vi "InitDrive.vi"   [LabVIEW 2019]
doc: "This VI initializes devices related directly to the drive subsystem."
uses:
  <vilib>/Rock Robotics/WPI/Solenoid/WPI_SolenoidChannel.ctl
  <vilib>/Rock Robotics/WPI/ThirdParty/Phoenix-LabVIEW/Motor Controller/Controls/CTRE_Phoenix_MotorControl_TalonFXInvertType.ctl
  <vilib>/Rock Robotics/WPI/ThirdParty/Phoenix-LabVIEW/Motor Controller/Controls/CTRE_Phoenix_MotorControl_NeutralMode.ctl
  <vilib>/Rock Robotics/WPI/ThirdParty/Phoenix-LabVIEW/Motor Controller/Controls/CTRE_Phoenix_MotorControl_SupplyCurrentLimitConfiguration.ctl
  <vilib>/Rock Robotics/WPI/ThirdParty/Phoenix-LabVIEW/Motor Controller/Controls/CTRE_Phoenix_MotorControl_FeedbackDevice_TalonFX.ctl
  <vilib>/Rock Robotics/WPI/Solenoid/WPI_SolenoidOpenDouble.vi
  refnums.vi
types:
  T1 = typedef "CTRE_Phoenix_MotorControl_TalonFXInvertType.ctl" = enum16{"Counter-Clockwise", "Clockwise"}
  T2 = typedef "CTRE_Phoenix_MotorControl_FeedbackDevice_TalonFX.ctl" = i8
  T3 = typedef "CTRE_Phoenix_MotorControl_SupplyCurrentLimitConfiguration.ctl" = cluster{"Enable?":bool, "Current Limit":dbl, "Threshold Current":dbl, "Threshold Time":dbl}
  T4 = typedef "CTRE_Phoenix_MotorControl_NeutralMode.ctl" = enum8{"EEPROMSetting", "Override to Coast", "Override to Brake"}
  T5 = typedef "WPI_SolenoidChannel.ctl" = enum8{"Solenoid 0", "Solenoid 1", "Solenoid 2", "Solenoid 3", "Solenoid 4", "Solenoid 5", "Solenoid 6", "Solenoid 7", "Invalid"}
  T6 = typedef "WPI_MotorControlDeviceRef.ctl" = cluster{"DeviceStatus":errorcluster, "Type":T7, "PWM":cluster{"PWM Channel":T8, "DeadBand":T9}, "CAN":cluster{"Device Number":u8, "SetOutput VI Ref":variant, "GetOutput VI Ref":variant, "Enable VI Ref":variant, "Disable VI Ref":variant, "Data":variant}, "Invert":bool, "DIO PWM":cluster{"PWM \"Enable\" Channel":T8, "DIOChannel":T10, "PWM Rate":dbl}}
  T7 = typedef "WPI_MotorControlType.ctl" = enum16{"PWM", "CAN", "DIO PWM"}
  T8 = typedef "FPGA_DIOPWMChannel.ctl" = enum8{"PWM 0", "PWM 1", "PWM 2", "PWM 3", "PWM 4", "PWM 5", "PWM 6", "PWM 7", "PWM 8", "PWM 9", "PWM MXP 0", "PWM MXP 1", "PWM MXP 2", "PWM MXP 3", "PWM MXP 4", "PWM MXP 5", "PWM MXP 6", "PWM MXP 7", "PWM MXP 8", "PWM MXP 9", "Invalid"}
  T9 = typedef "WPI_PWMDeadband.ctl" = cluster{"Name":string, "maxPositivePwm":i32, "minPositivePwm":i32, "centerPwm":i32, "maxNegativePwm":i32, "minNegativePwm":i32, "angularRange":u16}
  T10 = typedef "FPGA_DIOChannel.ctl" = enum8{"DIO 0", "DIO 1", "DIO 2", "DIO 3", "DIO 4", "DIO 5", "DIO 6", "DIO 7", "DIO 8", "DIO 9", "DIO MXP 0", "DIO MXP 1", "DIO MXP 2", "DIO MXP 3", "DIO MXP 4", "DIO MXP 5", "DIO MXP 6", "DIO MXP 7", "DIO MXP 8", "DIO MXP 9", "DIO MXP 10", "DIO MXP 11", "DIO MXP 12", "DIO MXP 13", "DIO MXP 14", "DIO MXP 15", "SPI Port CS1", "SPI Port CS2", "SPI Port CS3", "SPI Port MISO", "SPI Port MOSI", "Invalid"}
  T11 = typedef "WPI_SolenoidDevRef.ctl" = cluster{"DevStatus":errorcluster, "Pneumatics Control Module":u8, "Forward Solenoid Channel":T5, "Reverse Solenoid Channel":T5}
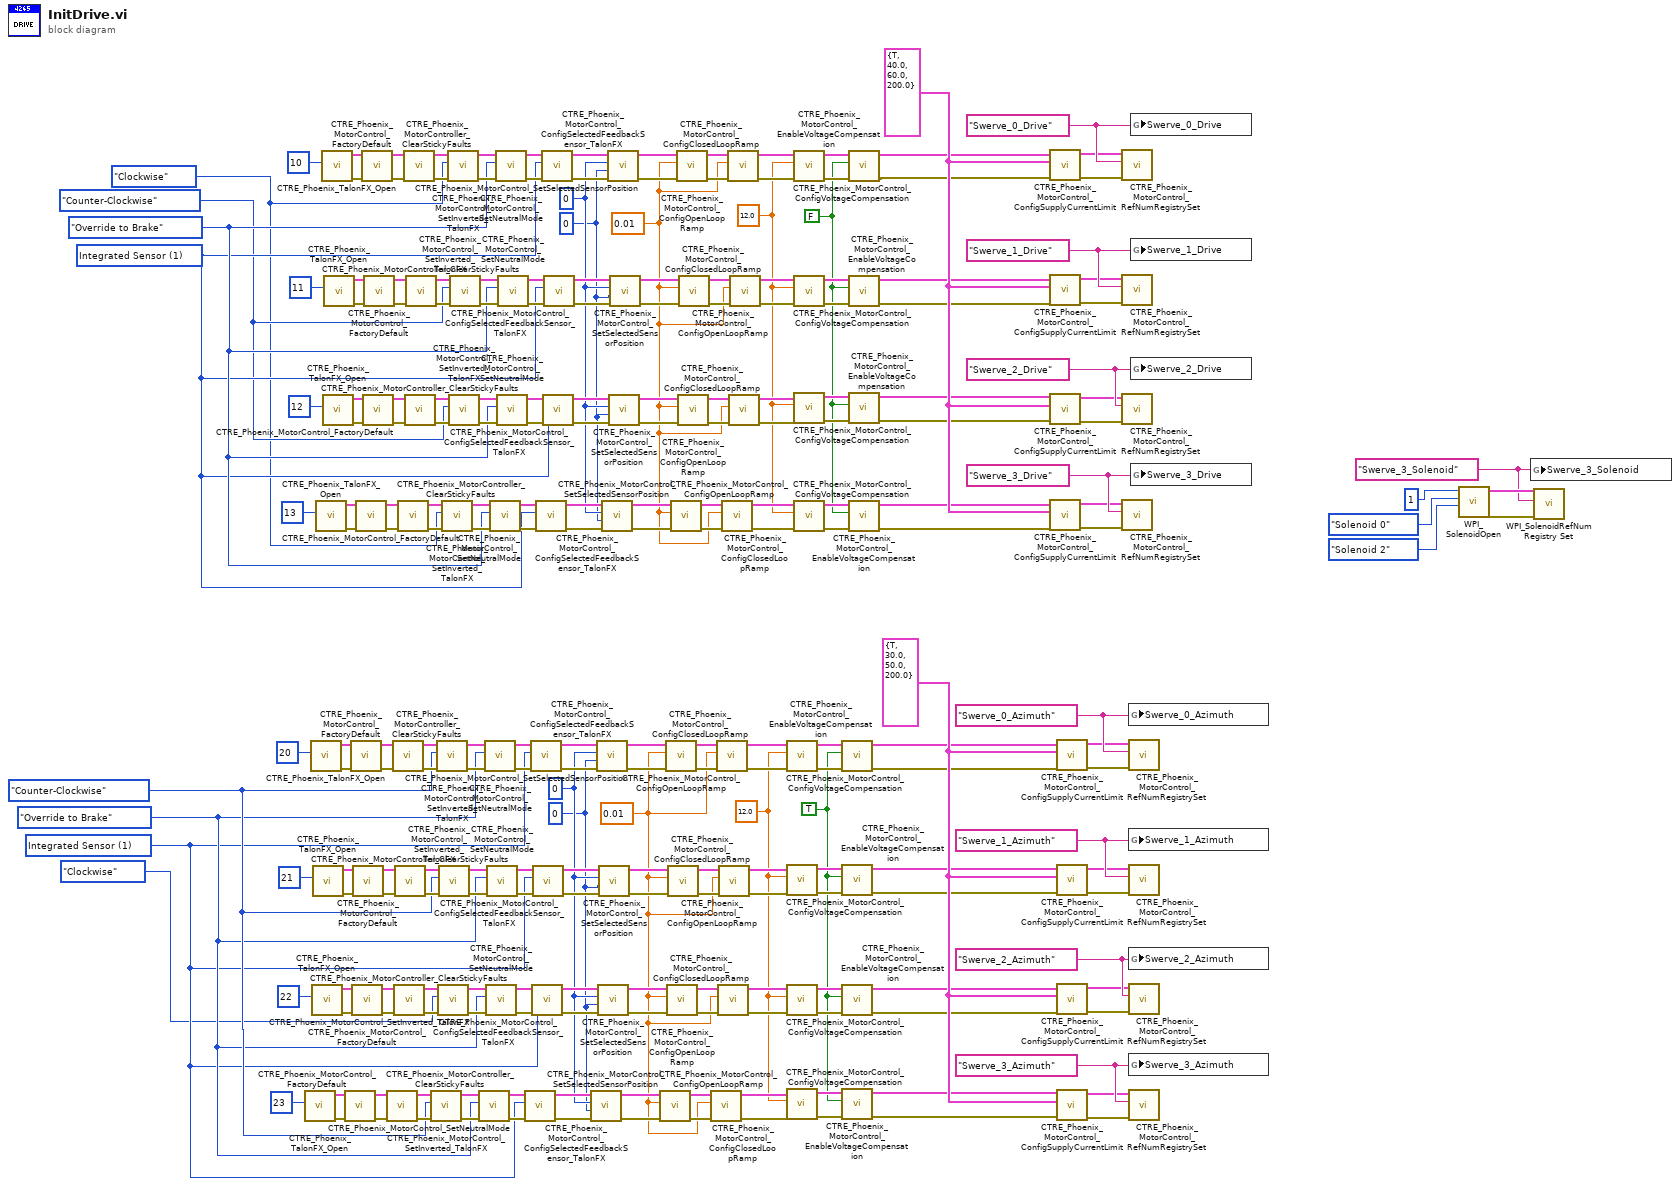
[diagram p0: block diagram]
diagram:
  w4 = CTRE_Phoenix_MotorControl_TalonFXInvertType."Clockwise" ("Invert Type")
  w6 = TRUE ("Enable Voltage Compensation?")
  w7 = 12.0 ("Saturation Voltage")
  w8 = FALSE ("Enable Voltage Compensation?")
  w9 = 12.0 ("Saturation Voltage")
  w56 = T2 1 items=["Integrated Sensor"=1, "Sensor Sum (S0 + S1)"=9, "Sensor Difference (D0 - D1)"=10, "Remote Source 0"=11, "Remote Source 1"=12, "None"=14, "Software Emulated"=15] ("Talon FX Feedback Device")
  w62 = T3 {"Enable?"=TRUE, "Current Limit"=30.0, "Threshold Current"=50.0, "Threshold Time"=200.0} ("Supply Current Limit Configuration")
  w57 = 0.01 ("secondsFromNeutralToFull")
  w58 = u32 0 ("pidLoopIdx")
  w59 = 0 ("New Sensor Position")
  w60 = CTRE_Phoenix_MotorControl_NeutralMode."Override to Brake" ("Motor Control Neutral Mode")
  w61 = CTRE_Phoenix_MotorControl_TalonFXInvertType."Counter-Clockwise" ("Invert Type")
  w78 = "Swerve_0_Azimuth" ("refnum name")
  w98 = "Swerve_1_Azimuth" ("refnum name")
  w118 = "Swerve_2_Azimuth" ("refnum name")
  w138 = "Swerve_3_Azimuth" ("refnum name")
  w146 = T2 1 items=["Integrated Sensor"=1, "Sensor Sum (S0 + S1)"=9, "Sensor Difference (D0 - D1)"=10, "Remote Source 0"=11, "Remote Source 1"=12, "None"=14, "Software Emulated"=15] ("Talon FX Feedback Device")
  w148 = T3 {"Enable?"=TRUE, "Current Limit"=40.0, "Threshold Current"=60.0, "Threshold Time"=200.0} ("Supply Current Limit Configuration")
  w143 = 0.01 ("secondsFromNeutralToFull")
  w144 = u32 0 ("pidLoopIdx")
  w145 = 0 ("New Sensor Position")
  w147 = CTRE_Phoenix_MotorControl_NeutralMode."Override to Brake" ("Motor Control Neutral Mode")
  w5 = CTRE_Phoenix_MotorControl_TalonFXInvertType."Counter-Clockwise" ("Invert Type")
  w164 = "Swerve_0_Drive" ("refnum name")
  w184 = "Swerve_1_Drive" ("refnum name")
  w204 = "Swerve_2_Drive" ("refnum name")
  w224 = "Swerve_3_Drive" ("refnum name")
  w229 = "Swerve_3_Solenoid" ("refnum name")
  n1 = call <vilib>:"CTRE_Phoenix_TalonFX_Open.vi"("Device Number"=u8 23 ("Drive 4L")) -> ("error out"=w127:errorcluster, "CAN Talon SRX Ref"=w134:T6)  [unwired: 9 in]
  n2 = call <vilib>:"CTRE_Phoenix_TalonFX_Open.vi"("Device Number"=u8 20 ("Drive 4L")) -> ("error out"=w67:errorcluster, "CAN Talon SRX Ref"=w74:T6)  [unwired: 9 in]
  n3 = call <vilib>:"CTRE_Phoenix_TalonFX_Open.vi"("Device Number"=u8 22 ("Drive 4L")) -> ("error out"=w107:errorcluster, "CAN Talon SRX Ref"=w114:T6)  [unwired: 9 in]
  n4 = call <vilib>:"CTRE_Phoenix_TalonFX_Open.vi"("Device Number"=u8 21 ("Drive 4L")) -> ("error out"=w87:errorcluster, "CAN Talon SRX Ref"=w94:T6)  [unwired: 9 in]
  n5 = call <vilib>:"CTRE_Phoenix_TalonFX_Open.vi"("Device Number"=u8 13 ("Drive 4L")) -> ("error out"=w213:errorcluster, "CAN Talon SRX Ref"=w220:T6)  [unwired: 9 in]
  n6 = call <vilib>:"CTRE_Phoenix_TalonFX_Open.vi"("Device Number"=u8 10 ("Drive 4L")) -> ("error out"=w153:errorcluster, "CAN Talon SRX Ref"=w160:T6)  [unwired: 9 in]
  n7 = call <vilib>:"CTRE_Phoenix_TalonFX_Open.vi"("Device Number"=u8 12 ("Drive 4L")) -> ("error out"=w193:errorcluster, "CAN Talon SRX Ref"=w200:T6)  [unwired: 9 in]
  n8 = call <vilib>:"CTRE_Phoenix_TalonFX_Open.vi"("Device Number"=u8 11 ("Drive 4L")) -> ("error out"=w173:errorcluster, "CAN Talon SRX Ref"=w180:T6)  [unwired: 9 in]
  n9 = call <vilib>:"CTRE_Phoenix_MotorControl_FactoryDefault.vi"("error in"=w127, "PhoenixMotorControlDevRef"=w134) -> ("error out"=w130:errorcluster, "PhoenixMotorControlDevRef"=w131:T6)  [unwired: 8 in]
  n10 = call <vilib>:"CTRE_Phoenix_MotorControl_FactoryDefault.vi"("error in"=w67, "PhoenixMotorControlDevRef"=w74) -> ("error out"=w70:errorcluster, "PhoenixMotorControlDevRef"=w71:T6)  [unwired: 8 in]
  n11 = call <vilib>:"CTRE_Phoenix_MotorControl_FactoryDefault.vi"("error in"=w107, "PhoenixMotorControlDevRef"=w114) -> ("error out"=w110:errorcluster, "PhoenixMotorControlDevRef"=w111:T6)  [unwired: 8 in]
  n12 = call <vilib>:"CTRE_Phoenix_MotorControl_FactoryDefault.vi"("error in"=w87, "PhoenixMotorControlDevRef"=w94) -> ("error out"=w90:errorcluster, "PhoenixMotorControlDevRef"=w91:T6)  [unwired: 8 in]
  n13 = call <vilib>:"CTRE_Phoenix_MotorControl_FactoryDefault.vi"("error in"=w213, "PhoenixMotorControlDevRef"=w220) -> ("error out"=w216:errorcluster, "PhoenixMotorControlDevRef"=w217:T6)  [unwired: 8 in]
  n14 = call <vilib>:"CTRE_Phoenix_MotorControl_FactoryDefault.vi"("error in"=w153, "PhoenixMotorControlDevRef"=w160) -> ("error out"=w156:errorcluster, "PhoenixMotorControlDevRef"=w157:T6)  [unwired: 8 in]
  n15 = call <vilib>:"CTRE_Phoenix_MotorControl_FactoryDefault.vi"("error in"=w193, "PhoenixMotorControlDevRef"=w200) -> ("error out"=w196:errorcluster, "PhoenixMotorControlDevRef"=w197:T6)  [unwired: 8 in]
  n16 = call <vilib>:"CTRE_Phoenix_MotorControl_FactoryDefault.vi"("error in"=w173, "PhoenixMotorControlDevRef"=w180) -> ("error out"=w176:errorcluster, "PhoenixMotorControlDevRef"=w177:T6)  [unwired: 8 in]
  n17 = call <vilib>:"CTRE_Phoenix_MotorController_ClearStickyFaults.vi"("error in"=w130, "PhoenixMotorControlDevRef"=w131) -> ("error out"=w129:errorcluster, "PhoenixMotorControlDevRef"=w128:T6)  [unwired: 8 in]
  n18 = call <vilib>:"CTRE_Phoenix_MotorController_ClearStickyFaults.vi"("error in"=w70, "PhoenixMotorControlDevRef"=w71) -> ("error out"=w69:errorcluster, "PhoenixMotorControlDevRef"=w68:T6)  [unwired: 8 in]
  n19 = call <vilib>:"CTRE_Phoenix_MotorController_ClearStickyFaults.vi"("error in"=w110, "PhoenixMotorControlDevRef"=w111) -> ("error out"=w109:errorcluster, "PhoenixMotorControlDevRef"=w108:T6)  [unwired: 8 in]
  n20 = call <vilib>:"CTRE_Phoenix_MotorController_ClearStickyFaults.vi"("error in"=w90, "PhoenixMotorControlDevRef"=w91) -> ("error out"=w89:errorcluster, "PhoenixMotorControlDevRef"=w88:T6)  [unwired: 8 in]
  n21 = call <vilib>:"CTRE_Phoenix_MotorController_ClearStickyFaults.vi"("error in"=w216, "PhoenixMotorControlDevRef"=w217) -> ("error out"=w215:errorcluster, "PhoenixMotorControlDevRef"=w214:T6)  [unwired: 8 in]
  n22 = call <vilib>:"CTRE_Phoenix_MotorController_ClearStickyFaults.vi"("error in"=w156, "PhoenixMotorControlDevRef"=w157) -> ("error out"=w155:errorcluster, "PhoenixMotorControlDevRef"=w154:T6)  [unwired: 8 in]
  n23 = call <vilib>:"CTRE_Phoenix_MotorController_ClearStickyFaults.vi"("error in"=w196, "PhoenixMotorControlDevRef"=w197) -> ("error out"=w195:errorcluster, "PhoenixMotorControlDevRef"=w194:T6)  [unwired: 8 in]
  n24 = call <vilib>:"CTRE_Phoenix_MotorController_ClearStickyFaults.vi"("error in"=w176, "PhoenixMotorControlDevRef"=w177) -> ("error out"=w175:errorcluster, "PhoenixMotorControlDevRef"=w174:T6)  [unwired: 8 in]
  n25 = call <vilib>:"CTRE_Phoenix_MotorControl_SetInverted_TalonFX.vi"("error in (no error)"=w129, "Invert Type"=w61, "PhoenixMotorControlDevRef"=w128) -> ("error out"=w141:errorcluster, "PhoenixMotorControlDevRef"=w142:T6)  [unwired: 7 in]
  n26 = call <vilib>:"CTRE_Phoenix_MotorControl_SetInverted_TalonFX.vi"("error in (no error)"=w69, "Invert Type"=w61, "PhoenixMotorControlDevRef"=w68) -> ("error out"=w81:errorcluster, "PhoenixMotorControlDevRef"=w82:T6)  [unwired: 7 in]
  n27 = call <vilib>:"CTRE_Phoenix_MotorControl_SetInverted_TalonFX.vi"("error in (no error)"=w109, "Invert Type"=CTRE_Phoenix_MotorControl_TalonFXInvertType."Clockwise", "PhoenixMotorControlDevRef"=w108) -> ("error out"=w121:errorcluster, "PhoenixMotorControlDevRef"=w122:T6)  [unwired: 7 in]
  n28 = call <vilib>:"CTRE_Phoenix_MotorControl_SetInverted_TalonFX.vi"("error in (no error)"=w89, "Invert Type"=w61, "PhoenixMotorControlDevRef"=w88) -> ("error out"=w101:errorcluster, "PhoenixMotorControlDevRef"=w102:T6)  [unwired: 7 in]
  n29 = call <vilib>:"CTRE_Phoenix_MotorControl_SetInverted_TalonFX.vi"("error in (no error)"=w215, "Invert Type"=w4, "PhoenixMotorControlDevRef"=w214) -> ("error out"=w227:errorcluster, "PhoenixMotorControlDevRef"=w228:T6)  [unwired: 7 in]
  n30 = call <vilib>:"CTRE_Phoenix_MotorControl_SetInverted_TalonFX.vi"("error in (no error)"=w155, "Invert Type"=w4, "PhoenixMotorControlDevRef"=w154) -> ("error out"=w167:errorcluster, "PhoenixMotorControlDevRef"=w168:T6)  [unwired: 7 in]
  n31 = call <vilib>:"CTRE_Phoenix_MotorControl_SetInverted_TalonFX.vi"("error in (no error)"=w195, "Invert Type"=w5, "PhoenixMotorControlDevRef"=w194) -> ("error out"=w207:errorcluster, "PhoenixMotorControlDevRef"=w208:T6)  [unwired: 7 in]
  n32 = call <vilib>:"CTRE_Phoenix_MotorControl_SetInverted_TalonFX.vi"("error in (no error)"=w175, "Invert Type"=w5, "PhoenixMotorControlDevRef"=w174) -> ("error out"=w187:errorcluster, "PhoenixMotorControlDevRef"=w188:T6)  [unwired: 7 in]
  n33 = call <vilib>:"CTRE_Phoenix_MotorControl_SetNeutralMode.vi"("error in (no error)"=w141, "Motor Control Neutral Mode"=w60, "PhoenixMotorControlDevRef"=w142) -> ("error out"=w125:errorcluster, "PhoenixMotorControlDevRef"=w126:T6)  [unwired: 7 in]
  n34 = call <vilib>:"CTRE_Phoenix_MotorControl_SetNeutralMode.vi"("error in (no error)"=w81, "Motor Control Neutral Mode"=w60, "PhoenixMotorControlDevRef"=w82) -> ("error out"=w65:errorcluster, "PhoenixMotorControlDevRef"=w66:T6)  [unwired: 7 in]
  n35 = call <vilib>:"CTRE_Phoenix_MotorControl_SetNeutralMode.vi"("error in (no error)"=w121, "Motor Control Neutral Mode"=w60, "PhoenixMotorControlDevRef"=w122) -> ("error out"=w105:errorcluster, "PhoenixMotorControlDevRef"=w106:T6)  [unwired: 7 in]
  n36 = call <vilib>:"CTRE_Phoenix_MotorControl_SetNeutralMode.vi"("error in (no error)"=w101, "Motor Control Neutral Mode"=w60, "PhoenixMotorControlDevRef"=w102) -> ("error out"=w85:errorcluster, "PhoenixMotorControlDevRef"=w86:T6)  [unwired: 7 in]
  n37 = call <vilib>:"CTRE_Phoenix_MotorControl_SetNeutralMode.vi"("error in (no error)"=w227, "Motor Control Neutral Mode"=w147, "PhoenixMotorControlDevRef"=w228) -> ("error out"=w211:errorcluster, "PhoenixMotorControlDevRef"=w212:T6)  [unwired: 7 in]
  n38 = call <vilib>:"CTRE_Phoenix_MotorControl_SetNeutralMode.vi"("error in (no error)"=w167, "Motor Control Neutral Mode"=w147, "PhoenixMotorControlDevRef"=w168) -> ("error out"=w151:errorcluster, "PhoenixMotorControlDevRef"=w152:T6)  [unwired: 7 in]
  n39 = call <vilib>:"CTRE_Phoenix_MotorControl_SetNeutralMode.vi"("error in (no error)"=w207, "Motor Control Neutral Mode"=w147, "PhoenixMotorControlDevRef"=w208) -> ("error out"=w191:errorcluster, "PhoenixMotorControlDevRef"=w192:T6)  [unwired: 7 in]
  n40 = call <vilib>:"CTRE_Phoenix_MotorControl_SetNeutralMode.vi"("error in (no error)"=w187, "Motor Control Neutral Mode"=w147, "PhoenixMotorControlDevRef"=w188) -> ("error out"=w171:errorcluster, "PhoenixMotorControlDevRef"=w172:T6)  [unwired: 7 in]
  n41 = call <vilib>:"CTRE_Phoenix_MotorControl_ConfigSelectedFeedbackSensor_TalonFX.vi"("error in (no error)"=w125, "Talon FX Feedback Device"=w56, "PhoenixMotorControlDevRef"=w126) -> ("error out"=w123:errorcluster, "PhoenixMotorControlDevRef"=w124:T6)  [unwired: 7 in]
  n42 = call <vilib>:"CTRE_Phoenix_MotorControl_ConfigSelectedFeedbackSensor_TalonFX.vi"("error in (no error)"=w65, "Talon FX Feedback Device"=w56, "PhoenixMotorControlDevRef"=w66) -> ("error out"=w63:errorcluster, "PhoenixMotorControlDevRef"=w64:T6)  [unwired: 7 in]
  n43 = call <vilib>:"CTRE_Phoenix_MotorControl_ConfigSelectedFeedbackSensor_TalonFX.vi"("error in (no error)"=w105, "Talon FX Feedback Device"=w56, "PhoenixMotorControlDevRef"=w106) -> ("error out"=w103:errorcluster, "PhoenixMotorControlDevRef"=w104:T6)  [unwired: 7 in]
  n44 = call <vilib>:"CTRE_Phoenix_MotorControl_ConfigSelectedFeedbackSensor_TalonFX.vi"("error in (no error)"=w85, "Talon FX Feedback Device"=w56, "PhoenixMotorControlDevRef"=w86) -> ("error out"=w83:errorcluster, "PhoenixMotorControlDevRef"=w84:T6)  [unwired: 7 in]
  n45 = call <vilib>:"CTRE_Phoenix_MotorControl_ConfigSelectedFeedbackSensor_TalonFX.vi"("error in (no error)"=w211, "Talon FX Feedback Device"=w146, "PhoenixMotorControlDevRef"=w212) -> ("error out"=w209:errorcluster, "PhoenixMotorControlDevRef"=w210:T6)  [unwired: 7 in]
  n46 = call <vilib>:"CTRE_Phoenix_MotorControl_ConfigSelectedFeedbackSensor_TalonFX.vi"("error in (no error)"=w151, "Talon FX Feedback Device"=w146, "PhoenixMotorControlDevRef"=w152) -> ("error out"=w149:errorcluster, "PhoenixMotorControlDevRef"=w150:T6)  [unwired: 7 in]
  n47 = call <vilib>:"CTRE_Phoenix_MotorControl_ConfigSelectedFeedbackSensor_TalonFX.vi"("error in (no error)"=w191, "Talon FX Feedback Device"=w146, "PhoenixMotorControlDevRef"=w192) -> ("error out"=w189:errorcluster, "PhoenixMotorControlDevRef"=w190:T6)  [unwired: 7 in]
  n48 = call <vilib>:"CTRE_Phoenix_MotorControl_ConfigSelectedFeedbackSensor_TalonFX.vi"("error in (no error)"=w171, "Talon FX Feedback Device"=w146, "PhoenixMotorControlDevRef"=w172) -> ("error out"=w169:errorcluster, "PhoenixMotorControlDevRef"=w170:T6)  [unwired: 7 in]
  n49 = call <vilib>:"CTRE_Phoenix_MotorControl_SetSelectedSensorPosition.vi"("error in (no error)"=w123, "pidLoopIdx"=w58, "New Sensor Position"=w59, "PhoenixMotorControlDevRef"=w124) -> ("error out"=w140:errorcluster, "PhoenixMotorControlDevRef"=w139:T6)  [unwired: 6 in]
  n50 = call <vilib>:"CTRE_Phoenix_MotorControl_SetSelectedSensorPosition.vi"("error in (no error)"=w63, "pidLoopIdx"=w58, "New Sensor Position"=w59, "PhoenixMotorControlDevRef"=w64) -> ("error out"=w80:errorcluster, "PhoenixMotorControlDevRef"=w79:T6)  [unwired: 6 in]
  n51 = call <vilib>:"CTRE_Phoenix_MotorControl_SetSelectedSensorPosition.vi"("error in (no error)"=w103, "pidLoopIdx"=w58, "New Sensor Position"=w59, "PhoenixMotorControlDevRef"=w104) -> ("error out"=w120:errorcluster, "PhoenixMotorControlDevRef"=w119:T6)  [unwired: 6 in]
  n52 = call <vilib>:"CTRE_Phoenix_MotorControl_SetSelectedSensorPosition.vi"("error in (no error)"=w83, "pidLoopIdx"=w58, "New Sensor Position"=w59, "PhoenixMotorControlDevRef"=w84) -> ("error out"=w100:errorcluster, "PhoenixMotorControlDevRef"=w99:T6)  [unwired: 6 in]
  n53 = call <vilib>:"CTRE_Phoenix_MotorControl_SetSelectedSensorPosition.vi"("error in (no error)"=w209, "pidLoopIdx"=w144, "New Sensor Position"=w145, "PhoenixMotorControlDevRef"=w210) -> ("error out"=w226:errorcluster, "PhoenixMotorControlDevRef"=w225:T6)  [unwired: 6 in]
  n54 = call <vilib>:"CTRE_Phoenix_MotorControl_SetSelectedSensorPosition.vi"("error in (no error)"=w149, "pidLoopIdx"=w144, "New Sensor Position"=w145, "PhoenixMotorControlDevRef"=w150) -> ("error out"=w166:errorcluster, "PhoenixMotorControlDevRef"=w165:T6)  [unwired: 6 in]
  n55 = call <vilib>:"CTRE_Phoenix_MotorControl_SetSelectedSensorPosition.vi"("error in (no error)"=w189, "pidLoopIdx"=w144, "New Sensor Position"=w145, "PhoenixMotorControlDevRef"=w190) -> ("error out"=w206:errorcluster, "PhoenixMotorControlDevRef"=w205:T6)  [unwired: 6 in]
  n56 = call <vilib>:"CTRE_Phoenix_MotorControl_SetSelectedSensorPosition.vi"("error in (no error)"=w169, "pidLoopIdx"=w144, "New Sensor Position"=w145, "PhoenixMotorControlDevRef"=w170) -> ("error out"=w186:errorcluster, "PhoenixMotorControlDevRef"=w185:T6)  [unwired: 6 in]
  n57 = call <vilib>:"CTRE_Phoenix_MotorControl_ConfigOpenLoopRamp.vi"("error in (no error)"=w140, "secondsFromNeutralToFull"=w57, "PhoenixMotorControlDevRef"=w139) -> ("error out"=w132:errorcluster, "PhoenixMotorControlDevRef"=w133:T6)  [unwired: 7 in]
  n58 = call <vilib>:"CTRE_Phoenix_MotorControl_ConfigOpenLoopRamp.vi"("error in (no error)"=w80, "secondsFromNeutralToFull"=w57, "PhoenixMotorControlDevRef"=w79) -> ("error out"=w72:errorcluster, "PhoenixMotorControlDevRef"=w73:T6)  [unwired: 7 in]
  n59 = call <vilib>:"CTRE_Phoenix_MotorControl_ConfigOpenLoopRamp.vi"("error in (no error)"=w120, "secondsFromNeutralToFull"=w57, "PhoenixMotorControlDevRef"=w119) -> ("error out"=w112:errorcluster, "PhoenixMotorControlDevRef"=w113:T6)  [unwired: 7 in]
  n60 = call <vilib>:"CTRE_Phoenix_MotorControl_ConfigOpenLoopRamp.vi"("error in (no error)"=w100, "secondsFromNeutralToFull"=w57, "PhoenixMotorControlDevRef"=w99) -> ("error out"=w92:errorcluster, "PhoenixMotorControlDevRef"=w93:T6)  [unwired: 7 in]
  n61 = call <vilib>:"CTRE_Phoenix_MotorControl_ConfigOpenLoopRamp.vi"("error in (no error)"=w226, "secondsFromNeutralToFull"=w143, "PhoenixMotorControlDevRef"=w225) -> ("error out"=w218:errorcluster, "PhoenixMotorControlDevRef"=w219:T6)  [unwired: 7 in]
  n62 = call <vilib>:"CTRE_Phoenix_MotorControl_ConfigOpenLoopRamp.vi"("error in (no error)"=w166, "secondsFromNeutralToFull"=w143, "PhoenixMotorControlDevRef"=w165) -> ("error out"=w158:errorcluster, "PhoenixMotorControlDevRef"=w159:T6)  [unwired: 7 in]
  n63 = call <vilib>:"CTRE_Phoenix_MotorControl_ConfigOpenLoopRamp.vi"("error in (no error)"=w206, "secondsFromNeutralToFull"=w143, "PhoenixMotorControlDevRef"=w205) -> ("error out"=w198:errorcluster, "PhoenixMotorControlDevRef"=w199:T6)  [unwired: 7 in]
  n64 = call <vilib>:"CTRE_Phoenix_MotorControl_ConfigOpenLoopRamp.vi"("error in (no error)"=w186, "secondsFromNeutralToFull"=w143, "PhoenixMotorControlDevRef"=w185) -> ("error out"=w178:errorcluster, "PhoenixMotorControlDevRef"=w179:T6)  [unwired: 7 in]
  n65 = call <vilib>:"CTRE_Phoenix_MotorControl_ConfigClosedLoopRamp.vi"("error in (no error)"=w132, "secondsFromNeutralToFull"=w57, "PhoenixMotorControlDevRef"=w133) -> ("error out"=w12:errorcluster, "PhoenixMotorControlDevRef"=w13:T6)  [unwired: 7 in]
  n66 = call <vilib>:"CTRE_Phoenix_MotorControl_ConfigClosedLoopRamp.vi"("error in (no error)"=w72, "secondsFromNeutralToFull"=w57, "PhoenixMotorControlDevRef"=w73) -> ("error out"=w24:errorcluster, "PhoenixMotorControlDevRef"=w25:T6)  [unwired: 7 in]
  n67 = call <vilib>:"CTRE_Phoenix_MotorControl_ConfigClosedLoopRamp.vi"("error in (no error)"=w112, "secondsFromNeutralToFull"=w57, "PhoenixMotorControlDevRef"=w113) -> ("error out"=w16:errorcluster, "PhoenixMotorControlDevRef"=w17:T6)  [unwired: 7 in]
  n68 = call <vilib>:"CTRE_Phoenix_MotorControl_ConfigClosedLoopRamp.vi"("error in (no error)"=w92, "secondsFromNeutralToFull"=w57, "PhoenixMotorControlDevRef"=w93) -> ("error out"=w20:errorcluster, "PhoenixMotorControlDevRef"=w21:T6)  [unwired: 7 in]
  n69 = call <vilib>:"CTRE_Phoenix_MotorControl_ConfigClosedLoopRamp.vi"("error in (no error)"=w218, "secondsFromNeutralToFull"=w143, "PhoenixMotorControlDevRef"=w219) -> ("error out"=w28:errorcluster, "PhoenixMotorControlDevRef"=w29:T6)  [unwired: 7 in]
  n70 = call <vilib>:"CTRE_Phoenix_MotorControl_ConfigClosedLoopRamp.vi"("error in (no error)"=w158, "secondsFromNeutralToFull"=w143, "PhoenixMotorControlDevRef"=w159) -> ("error out"=w38:errorcluster, "PhoenixMotorControlDevRef"=w39:T6)  [unwired: 7 in]
  n71 = call <vilib>:"CTRE_Phoenix_MotorControl_ConfigClosedLoopRamp.vi"("error in (no error)"=w198, "secondsFromNeutralToFull"=w143, "PhoenixMotorControlDevRef"=w199) -> ("error out"=w32:errorcluster, "PhoenixMotorControlDevRef"=w33:T6)  [unwired: 7 in]
  n72 = call <vilib>:"CTRE_Phoenix_MotorControl_ConfigClosedLoopRamp.vi"("error in (no error)"=w178, "secondsFromNeutralToFull"=w143, "PhoenixMotorControlDevRef"=w179) -> ("error out"=w36:errorcluster, "PhoenixMotorControlDevRef"=w37:T6)  [unwired: 7 in]
  n73 = call <vilib>:"CTRE_Phoenix_MotorControl_ConfigVoltageCompensation.vi"("error in (no error)"=w24, "Saturation Voltage"=w7, "PhoenixMotorControlDevRef"=w25) -> ("error out"=w46:errorcluster, "PhoenixMotorControlDevRef"=w47:T6)  [unwired: 7 in]
  n74 = call <vilib>:"CTRE_Phoenix_MotorControl_ConfigVoltageCompensation.vi"("error in (no error)"=w20, "Saturation Voltage"=w7, "PhoenixMotorControlDevRef"=w21) -> ("error out"=w44:errorcluster, "PhoenixMotorControlDevRef"=w45:T6)  [unwired: 7 in]
  n75 = call <vilib>:"CTRE_Phoenix_MotorControl_ConfigVoltageCompensation.vi"("error in (no error)"=w16, "Saturation Voltage"=w7, "PhoenixMotorControlDevRef"=w17) -> ("error out"=w42:errorcluster, "PhoenixMotorControlDevRef"=w43:T6)  [unwired: 7 in]
  n76 = call <vilib>:"CTRE_Phoenix_MotorControl_ConfigVoltageCompensation.vi"("error in (no error)"=w12, "Saturation Voltage"=w7, "PhoenixMotorControlDevRef"=w13) -> ("error out"=w40:errorcluster, "PhoenixMotorControlDevRef"=w41:T6)  [unwired: 7 in]
  n77 = call <vilib>:"CTRE_Phoenix_MotorControl_ConfigVoltageCompensation.vi"("error in (no error)"=w38, "Saturation Voltage"=w9, "PhoenixMotorControlDevRef"=w39) -> ("error out"=w54:errorcluster, "PhoenixMotorControlDevRef"=w55:T6)  [unwired: 7 in]
  n78 = call <vilib>:"CTRE_Phoenix_MotorControl_ConfigVoltageCompensation.vi"("error in (no error)"=w36, "Saturation Voltage"=w9, "PhoenixMotorControlDevRef"=w37) -> ("error out"=w52:errorcluster, "PhoenixMotorControlDevRef"=w53:T6)  [unwired: 7 in]
  n79 = call <vilib>:"CTRE_Phoenix_MotorControl_ConfigVoltageCompensation.vi"("error in (no error)"=w32, "Saturation Voltage"=w9, "PhoenixMotorControlDevRef"=w33) -> ("error out"=w50:errorcluster, "PhoenixMotorControlDevRef"=w51:T6)  [unwired: 7 in]
  n80 = call <vilib>:"CTRE_Phoenix_MotorControl_ConfigVoltageCompensation.vi"("error in (no error)"=w28, "Saturation Voltage"=w9, "PhoenixMotorControlDevRef"=w29) -> ("error out"=w48:errorcluster, "PhoenixMotorControlDevRef"=w49:T6)  [unwired: 7 in]
  n81 = call <vilib>:"CTRE_Phoenix_MotorControl_EnableVoltageCompensation.vi"("error in (no error)"=w46, "Enable Voltage Compensation?"=w6, "PhoenixMotorControlDevRef"=w47) -> ("error out"=w22:errorcluster, "PhoenixMotorControlDevRef"=w23:T6)  [unwired: 7 in]
  n82 = call <vilib>:"CTRE_Phoenix_MotorControl_EnableVoltageCompensation.vi"("error in (no error)"=w44, "Enable Voltage Compensation?"=w6, "PhoenixMotorControlDevRef"=w45) -> ("error out"=w18:errorcluster, "PhoenixMotorControlDevRef"=w19:T6)  [unwired: 7 in]
  n83 = call <vilib>:"CTRE_Phoenix_MotorControl_EnableVoltageCompensation.vi"("error in (no error)"=w42, "Enable Voltage Compensation?"=w6, "PhoenixMotorControlDevRef"=w43) -> ("error out"=w14:errorcluster, "PhoenixMotorControlDevRef"=w15:T6)  [unwired: 7 in]
  n84 = call <vilib>:"CTRE_Phoenix_MotorControl_EnableVoltageCompensation.vi"("error in (no error)"=w40, "Enable Voltage Compensation?"=w6, "PhoenixMotorControlDevRef"=w41) -> ("error out"=w10:errorcluster, "PhoenixMotorControlDevRef"=w11:T6)  [unwired: 7 in]
  n85 = call <vilib>:"CTRE_Phoenix_MotorControl_EnableVoltageCompensation.vi"("error in (no error)"=w54, "Enable Voltage Compensation?"=w8, "PhoenixMotorControlDevRef"=w55) -> ("error out"=w1:errorcluster, "PhoenixMotorControlDevRef"=w2:T6)  [unwired: 7 in]
  n86 = call <vilib>:"CTRE_Phoenix_MotorControl_EnableVoltageCompensation.vi"("error in (no error)"=w52, "Enable Voltage Compensation?"=w8, "PhoenixMotorControlDevRef"=w53) -> ("error out"=w34:errorcluster, "PhoenixMotorControlDevRef"=w35:T6)  [unwired: 7 in]
  n87 = call <vilib>:"CTRE_Phoenix_MotorControl_EnableVoltageCompensation.vi"("error in (no error)"=w50, "Enable Voltage Compensation?"=w8, "PhoenixMotorControlDevRef"=w51) -> ("error out"=w30:errorcluster, "PhoenixMotorControlDevRef"=w31:T6)  [unwired: 7 in]
  n88 = call <vilib>:"CTRE_Phoenix_MotorControl_EnableVoltageCompensation.vi"("error in (no error)"=w48, "Enable Voltage Compensation?"=w8, "PhoenixMotorControlDevRef"=w49) -> ("error out"=w26:errorcluster, "PhoenixMotorControlDevRef"=w27:T6)  [unwired: 7 in]
  n89 = call <vilib>:"CTRE_Phoenix_MotorControl_ConfigSupplyCurrentLimit.vi"("error in (no error)"=w1, "Supply Current Limit Configuration"=w148, "PhoenixMotorControlDevRef"=w2) -> ("error out"=w162:errorcluster, "PhoenixMotorControlDevRef"=w163:T6)  [unwired: 7 in]
  n90 = call <vilib>:"CTRE_Phoenix_MotorControl_ConfigSupplyCurrentLimit.vi"("error in (no error)"=w34, "Supply Current Limit Configuration"=w148, "PhoenixMotorControlDevRef"=w35) -> ("error out"=w182:errorcluster, "PhoenixMotorControlDevRef"=w183:T6)  [unwired: 7 in]
  n91 = call <vilib>:"CTRE_Phoenix_MotorControl_ConfigSupplyCurrentLimit.vi"("error in (no error)"=w30, "Supply Current Limit Configuration"=w148, "PhoenixMotorControlDevRef"=w31) -> ("error out"=w202:errorcluster, "PhoenixMotorControlDevRef"=w203:T6)  [unwired: 7 in]
  n92 = call <vilib>:"CTRE_Phoenix_MotorControl_ConfigSupplyCurrentLimit.vi"("error in (no error)"=w26, "Supply Current Limit Configuration"=w148, "PhoenixMotorControlDevRef"=w27) -> ("error out"=w222:errorcluster, "PhoenixMotorControlDevRef"=w223:T6)  [unwired: 7 in]
  n93 = call <vilib>:"CTRE_Phoenix_MotorControl_ConfigSupplyCurrentLimit.vi"("error in (no error)"=w22, "Supply Current Limit Configuration"=w62, "PhoenixMotorControlDevRef"=w23) -> ("error out"=w76:errorcluster, "PhoenixMotorControlDevRef"=w77:T6)  [unwired: 7 in]
  n94 = call <vilib>:"CTRE_Phoenix_MotorControl_ConfigSupplyCurrentLimit.vi"("error in (no error)"=w18, "Supply Current Limit Configuration"=w62, "PhoenixMotorControlDevRef"=w19) -> ("error out"=w96:errorcluster, "PhoenixMotorControlDevRef"=w97:T6)  [unwired: 7 in]
  n95 = call <vilib>:"CTRE_Phoenix_MotorControl_ConfigSupplyCurrentLimit.vi"("error in (no error)"=w14, "Supply Current Limit Configuration"=w62, "PhoenixMotorControlDevRef"=w15) -> ("error out"=w116:errorcluster, "PhoenixMotorControlDevRef"=w117:T6)  [unwired: 7 in]
  n96 = call <vilib>:"CTRE_Phoenix_MotorControl_ConfigSupplyCurrentLimit.vi"("error in (no error)"=w10, "Supply Current Limit Configuration"=w62, "PhoenixMotorControlDevRef"=w11) -> ("error out"=w136:errorcluster, "PhoenixMotorControlDevRef"=w137:T6)  [unwired: 7 in]
  n97 = call <vilib>:"CTRE_Phoenix_MotorControl_RefNumRegistrySet.vi"("error in (no error)"=w162, "refnum name"=w164, "PhoenixMotorControlDevRef"=w163) -> ()  [unwired: 7 in, 2 out]
  n98 = call <vilib>:"CTRE_Phoenix_MotorControl_RefNumRegistrySet.vi"("error in (no error)"=w182, "refnum name"=w184, "PhoenixMotorControlDevRef"=w183) -> ()  [unwired: 7 in, 2 out]
  n99 = call <vilib>:"CTRE_Phoenix_MotorControl_RefNumRegistrySet.vi"("error in (no error)"=w202, "refnum name"=w204, "PhoenixMotorControlDevRef"=w203) -> ()  [unwired: 7 in, 2 out]
  n100 = call <vilib>:"CTRE_Phoenix_MotorControl_RefNumRegistrySet.vi"("error in (no error)"=w222, "refnum name"=w224, "PhoenixMotorControlDevRef"=w223) -> ()  [unwired: 7 in, 2 out]
  n101 = global write "refnums.vi" "Swerve_0_Azimuth"(w78) -> ()
  n102 = call <vilib>:"CTRE_Phoenix_MotorControl_RefNumRegistrySet.vi"("error in (no error)"=w76, "refnum name"=w78, "PhoenixMotorControlDevRef"=w77) -> ()  [unwired: 7 in, 2 out]
  n103 = global write "refnums.vi" "Swerve_1_Azimuth"(w98) -> ()
  n104 = call <vilib>:"CTRE_Phoenix_MotorControl_RefNumRegistrySet.vi"("error in (no error)"=w96, "refnum name"=w98, "PhoenixMotorControlDevRef"=w97) -> ()  [unwired: 7 in, 2 out]
  n105 = global write "refnums.vi" "Swerve_2_Azimuth"(w118) -> ()
  n106 = call <vilib>:"CTRE_Phoenix_MotorControl_RefNumRegistrySet.vi"("error in (no error)"=w116, "refnum name"=w118, "PhoenixMotorControlDevRef"=w117) -> ()  [unwired: 7 in, 2 out]
  n107 = global write "refnums.vi" "Swerve_3_Azimuth"(w138) -> ()
  n108 = call <vilib>:"CTRE_Phoenix_MotorControl_RefNumRegistrySet.vi"("error in (no error)"=w136, "refnum name"=w138, "PhoenixMotorControlDevRef"=w137) -> ()  [unwired: 7 in, 2 out]
  n109 = global write "refnums.vi" "Swerve_0_Drive"(w164) -> ()
  n110 = global write "refnums.vi" "Swerve_1_Drive"(w184) -> ()
  n111 = global write "refnums.vi" "Swerve_2_Drive"(w204) -> ()
  n112 = global write "refnums.vi" "Swerve_3_Drive"(w224) -> ()
  n113 = call-poly <vilib>:"WPI_SolenoidOpen.vi"("Reverse Solenoid Channel"=WPI_SolenoidChannel."Solenoid 2", "Forward Solenoid Channel"=WPI_SolenoidChannel."Solenoid 0", "Pneumatics Control Module (0)"=u8 1) -> ("error out"=w230:errorcluster, "SolenoidDevRef"=w231:T11)  [unwired: 7 in]
  n114 = global write "refnums.vi" "Swerve_3_Solenoid"(w229) -> ()
  n115 = call <vilib>:"WPI_SolenoidRefNum Registry Set.vi"("error in (no error)"=w230, "refnum name"=w229, "SolenoidDevRef"=w231) -> ()  [unwired: 7 in, 2 out]
